vi "test CANopen AF.vi"() -> ()   [LabVIEW 2024]
uses:
  CANopen Test UI/CANopen Test UI/CANopen Test UI Actor.lvclass
  <vilib>/ActorFramework/Actor/Actor.lvclass
  C:/Program Files/National Instruments/LabVIEW 2024/vi.lib/ActorFramework/Actor/Actor.lvclass
  D:/git/CANopen-XNET/CANopen Test UI/CANopen Test UI/CANopen Test UI Actor.lvclass
panel:
  out "error out":errorcluster
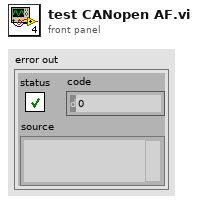
[diagram p1: front panel]
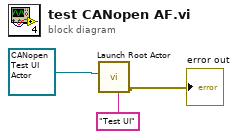
[diagram p0: block diagram]
diagram:
  n1 = call <vilib>:"Launch Root Actor.vi"("Debug Alias"="Test UI", "Actor"=refnum<class "CANopen Test UI Actor.lvclass"> refnum ("CANopen Test UI.lvlib:CANopen Test UI.lvclass")) -> ("error out"=→"error out":errorcluster)  [unwired: 8 in, 1 out]
